vi "RS-232A.vi"(0 "bytes to read":u32=5, 2 "Verify CheckSum":bool=TRUE, 3 "Read COM Port":bool=TRUE, 5 "String To Write":string="*IDN?", 6 "Add CheckSum":bool=TRUE, 7 "Write to COM Port":bool=TRUE, 8 "Close COMPort":bool=TRUE, 9 "Initialize COMPort":bool=TRUE, 10 "baud rate":u32=9600, 11 "VISA resource name":refnum<visa-resource-name>="COM1") -> (1 "OK?":bool, 4 "Read String":string)   [LabVIEW 2014]
doc: "The Basic Serial Read and Write example performs a Serial Port Read, a Serial Port Write, or a combination of these actions. The user selects the actions (read or write) on the front panel. If both are selected, the VI will write the data first, read data, and then close the VISA session that is opened to the port. This VI will wait until the specified number of bytes is received at the port. Only the number of bytes specified will be read.\n\nINSTRUCTIONS:\n1) Select the serial resource and configuration parameters (baud rate, data bits, parity, stop bits, flow control).\n2) Select the operations to be performed. \n3) Connect the serial port to your device. If no device is available, perform a loopback test by doing one of the following. Short pins 2 and 3 on a RS-232 cable or short pin 4 to pin 8 and pin 5 to pin 9 on a RS-485/422 cable. \n4) Run the VI to see the data read. (The \"read string\" will match the \"string to write\" if a loopback test was performed.)\n\nNote: The parameters set for the serial port must match the parameters of the connected instrument or device. In this example, the bytes to read parameter specifies the number of bytes that the serial port reads. If there were more bytes at the port than the number specified in bytes to read, those bytes would not be read. Also, if you specify to read more bytes than the number of bytes actually read, you might receive a timeout error message.\n\nOn the block diagram, the Configure Serial Port VI sets the configuration parameters. The front panel displays the controls used to configure the basic parameters, such as baud rate, data bits, and parity. Constants configure the other parameters the user probably does not need set. After the VISA Configure Serial Port VI opens the VISA session and configures the port, the VI passes the VISA resource name to other VIs that perform operations on that VISA resource. The VISA Write function sends a command to the serial device and the VISA Read function returns data based on the command. The VISA Close function then closes the reference to the serial device. It is important to close the reference; otherwise communication through with that port through protocols other than VISA might not be possible."
uses:
  <vilib>/Instr/_visa.llb/VISA Configure Serial Port (Instr).vi
panel:
  in  "flow control":u16(ring) items=["None"=0, "XON/XOFF"=1, "RTS/CTS"=2, "DTR/DSR"=4]
  in  "stop bits":u16(ring)=10 items=["1.0"=10, "1.5"=15, "2.0"=20]
  in  "parity":u16(ring) items=["None", "Odd", "Even", "Mark", "Space"]
  in  "data bits":u16=8 min=5 max=8 step=1
  # "Select the serial resource and the operations (Read, Write, or both) to be performed.  If both are selected, the VI will write the data first, read data and then close the VISA session that is opened to the port.  This VI will wait until the specified number of bytes is received at the port. Only the number of bytes specified will be read."
  # "For additional information select File >> VI Properties >> Documentation"
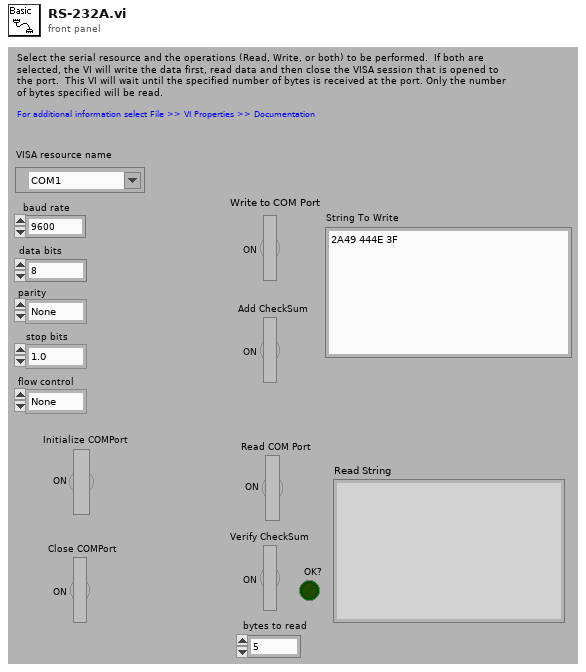
[diagram p1: front panel]
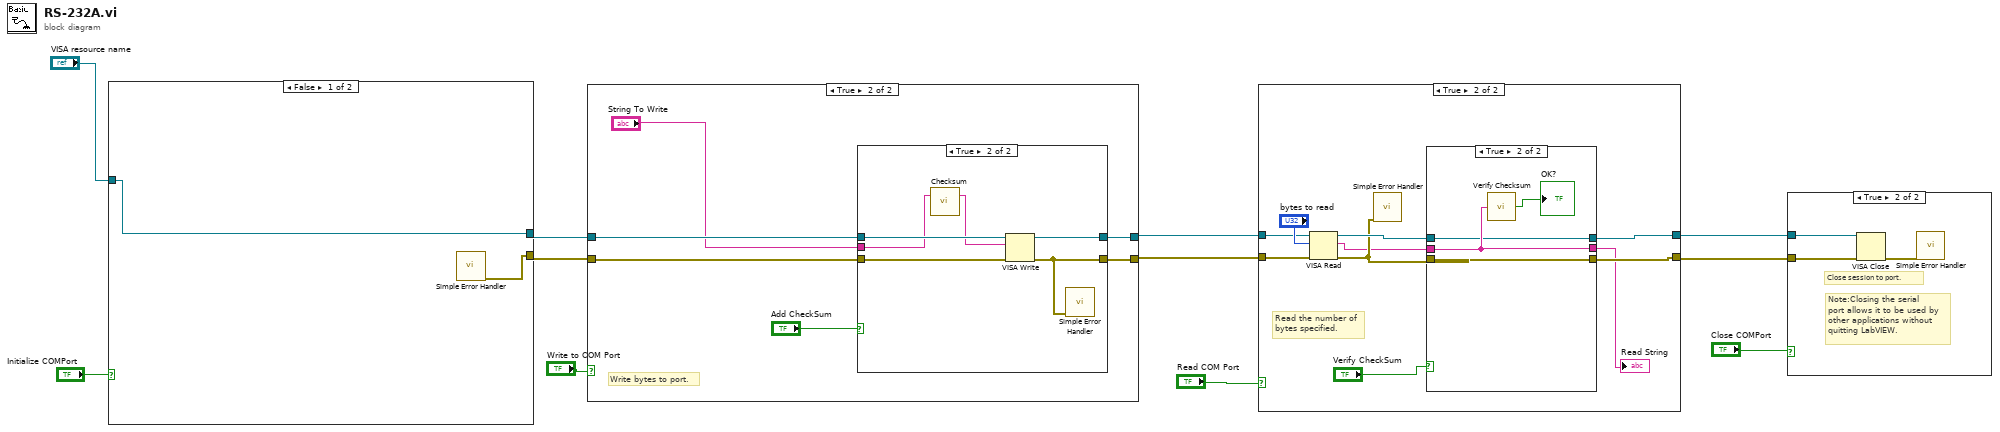
[diagram p0: block diagram]
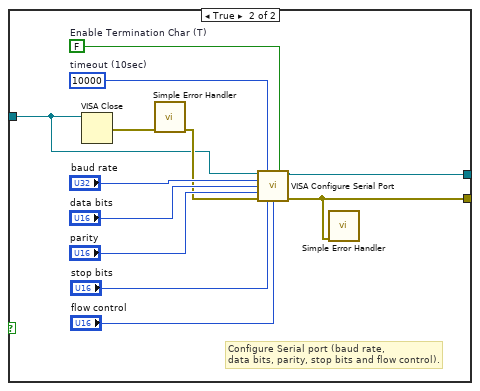
[diagram p3: hidden frame]
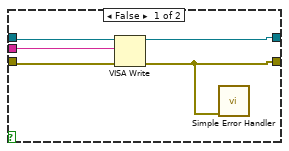
[diagram p5: hidden frame]
diagram:
  n1 = case shown="False" "Initialize COMPort" {
    tunnel: "VISA resource name" -> [w13 w15]
    tunnel: [w13 w18] -> w3
    tunnel: [w12 w14] -> w2
    frame False {
      n2 = call <vilib>:"Simple Error Handler.vi"() -> ("error out"=w12:errorcluster)  [unwired: 5 in, 4 out]
    }
    frame True {
      w22 = FALSE  # Enable Termination Char (T)
      w23 = u32 10000  # timeout (10sec)
      # "Configure Serial port (baud rate,\ndata bits, parity, stop bits and flow control)."
      n3 = VISA Close(VISA resource name=w15) -> (error out=w17:errorcluster)  [unwired: 1 in]
      n4 = call <vilib>:"Simple Error Handler.vi"("error in (no error)"=w17) -> ("error out"=w16:errorcluster)  [unwired: 4 in, 4 out]
      n5 = call-poly "VISA Configure Serial Port"("VISA resource name"=w15, "timeout (10sec)"=w23, "Enable Termination\nChar (T)"=w22, "baud rate (9600)"="baud rate", "data bits (8)"="data bits", "parity (0:none)"="parity", "error in (no error)"=w16, "stop bits (10: 1 bit)"="stop bits", "flow control (0:none)"="flow control") -> ("VISA resource name out"=w18:refnum<visa-resource-name>, "error out"=w14:errorcluster)  [unwired: 5 in]
      n6 = call <vilib>:"Simple Error Handler.vi"("error in (no error)"=w14) -> ()  [unwired: 4 in, 5 out]
    }
  }
  n7 = case shown="True" "Write to COM Port" {
    tunnel: [w27 w33] -> w10
    tunnel: w3 -> [w26 w32]
    tunnel: w2 -> [w27 w31]
    tunnel: [w26 w30] -> w6
    frame False {
    }
    frame True {
      # "Write bytes to port."
      n8 = case shown="True" "Add CheckSum" {
        tunnel: [w34 w39] -> w33
        tunnel: w32 -> [w37 w44]
        tunnel: w31 -> [w36 w43]
        tunnel: [w38 w42] -> w30
        tunnel: "String To Write" -> [w35 w41]
        frame False {
          n9 = VISA Write(VISA resource name=w37, write buffer=w35, error in (no error)=w36) -> (VISA resource name out=w38:refnum<visa-resource-name>, error out=w34:errorcluster)  [unwired: 1 out]
          n10 = call <vilib>:"Simple Error Handler.vi"("error in (no error)"=w34) -> ()  [unwired: 4 in, 5 out]
        }
        frame True {
          n11 = call "Checksum.vi"("HEX String to Calculate CheckSum"=w41) -> ("Hex String with CheckSum"=w40:string)  [unwired: 2 out]
          n12 = VISA Write(VISA resource name=w44, write buffer=w40, error in (no error)=w43) -> (VISA resource name out=w42:refnum<visa-resource-name>, error out=w39:errorcluster)  [unwired: 1 out]
          n13 = call <vilib>:"Simple Error Handler.vi"("error in (no error)"=w39) -> ()  [unwired: 4 in, 5 out]
        }
      }
    }
  }
  n14 = case shown="True" "Read COM Port" {
    tunnel: w10 -> [w46 w55]
    tunnel: [w46 w49] -> w9
    tunnel: [w45 w51] -> w8
    tunnel: w6 -> [w45 w54]
    frame False {
    }
    frame True {
      # "Read the number of bytes specified."
      n15 = VISA Read(VISA resource name=w54, byte count="bytes to read", error in (no error)=w55) -> (VISA resource name out=w52:refnum<visa-resource-name>, read buffer=w48:string, error out=w50:errorcluster)  [unwired: 1 out]
      n16 = call <vilib>:"Simple Error Handler.vi"("error in (no error)"=w50) -> ()  [unwired: 4 in, 5 out]
      n17 = case shown="True" "Verify CheckSum" {
        tunnel: w52 -> [w59 w61]
        tunnel: [w59 w61] -> w51
        tunnel: w50 -> [w58 w60]
        tunnel: [w58 w60] -> w49
        tunnel: w48 -> [w57 w63]
        tunnel: [w57 w63] -> w47
        frame False {
        }
        frame True {
          n18 = call "Verify Checksum.vi"("HEX String to Verify CheckSum"=w63) -> ("CheckSum OK"=→"OK?":bool)
        }
      }
      "Read String" <- w47
    }
  }
  n19 = case shown="True" "Close COMPort" {
    tunnel: w9 -> [_ w66]
    tunnel: w8 -> [_ w65]
    frame False {
    }
    frame True {
      # "Note:Closing the serial port allows it to be used by other applications without\nquitting LabVIEW."
      # "Close session to port."
      n20 = VISA Close(VISA resource name=w65, error in (no error)=w66) -> (error out=w64:errorcluster)
      n21 = call <vilib>:"Simple Error Handler.vi"("error in (no error)"=w64) -> ()  [unwired: 4 in, 5 out]
    }
  }
